vi "System Read String.vi"(8 "error in (no error)":errorcluster {"code" format="%.0x"}, 9 "ValBufferSize":i32=256, 11 "instrument handle":refnum<k15>) -> (0 "error out":errorcluster {"code" format="%.0x"}, 2 "Val":string, 3 "instrument handle out":refnum<k15>)   [LabVIEW 2021, in "Keysight XSAnVMA.lvlib"]
doc: "Reads a complete response from the instrument and returns it as a string."
uses:
  <instrlib>/Keysight XSAnVMA/Keysight XSAnVMA.lvlib
  KtXSAnVMA_64.dll
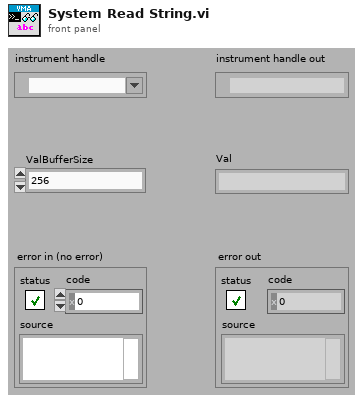
[diagram p1: front panel]
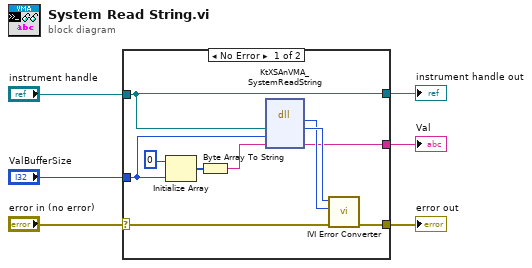
[diagram p0: block diagram]
diagram:
  n1 = case shown="No Error" "error in (no error)" {
    selector: "error in (no error)" -> [w14 w18]
    tunnel: [w13 w18] -> w6
    tunnel: "instrument handle" -> [w8 w17]
    tunnel: "ValBufferSize" -> [w7 _]
    tunnel: [w9 _] -> w2
    tunnel: [w8 w17] -> w1
    frame No Error {
      n2 = Initialize Array(u8 0 ("element"), w7) -> (w11:u8[])
      n3 = Byte Array To String(unsigned byte array=w11) -> (string=w12:string)
      n4 = dll-call lib="KtXSAnVMA**.dll" fn="KtXSAnVMA_SystemReadString"("Vi"=w8, "ValBufferSize"=w7, "Val"=w12) -> (w15:i32, "Vi"=w16:u32, "Val"=w9:string)  [unwired: 4 in, 2 out]
      n5 = call <instrlib>:"IVI Error Converter.vi"("error in (no error)"=w14, "IVI error code (0)"=w15, "instrument handle"=w16) -> ("error out"=w13:errorcluster)  [unwired: 7 in, 1 out]
    }
    frame Error {
    }
  }
  "error out" <- w6
  "instrument handle out" <- w1
  "Val" <- w2
